vi "provePilot.vi"(8 "error in":errorcluster, 9 "Boiler Simulation Controls":refnum<vi>, 10 "Boiler Controls":refnum<vi>, 11 "Boiler Status Indicators":refnum<vi>) -> (0 "error out":errorcluster, 3 "sensor":dbl)   [LabVIEW 2024]
uses:
  Controls/Boiler Simulation Controls.ctl
  Controls/Boiler Status Indicators.ctl
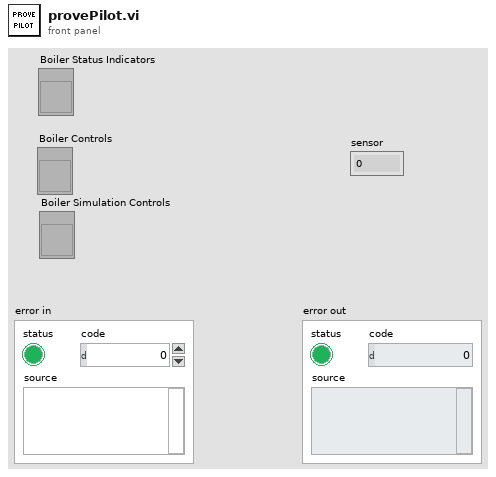
[diagram p1: front panel]
types:
  T1 = typedef "Boiler Simulation Controls.ctl" = cluster{"Flame Sensor Value (%)":dbl, "Run Interlock":bool, "Forced Draft Fan":bool}
  T2 = typedef "Boiler Status Indicators.ctl" = cluster{"Status":string, "Primary Fan":bool, "Natural Gas Valve":bool, "Pilot":bool, "Fuel Valve":bool, "Forced Draft Fan":bool, "Time Count":dbl}
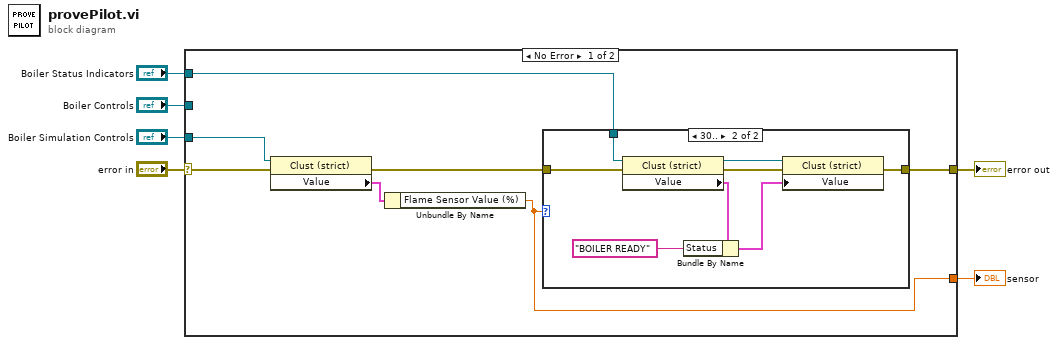
[diagram p0: block diagram]
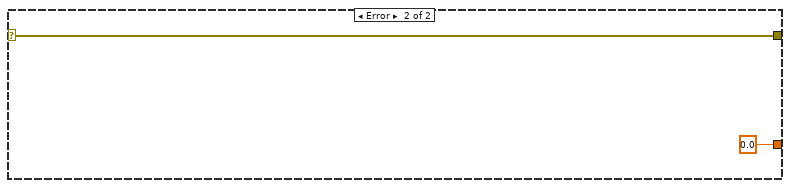
[diagram p3: hidden frame]
diagram:
  n1 = case shown="No Error" "error in" {
    selector: "error in" -> [w12 w24]
    tunnel: [w8 w24] -> w5
    tunnel: "Boiler Status Indicators" -> [w13 _]
    tunnel: [w7 0.0] -> w3
    tunnel: "Boiler Controls" -> [_ _]
    tunnel: "Boiler Simulation Controls" -> [w10 _]
    frame No Error {
      n2 = property class="Clust (strict)"(reference=w10, error in=w12) -> (error out=w11:errorcluster, "Value"=w9:T1)  [unwired: 1 out]
      n3 = Unbundle By Name(w9) -> ("Flame Sensor Value (%)"=w7:dbl)
      n4 = case shown="30.." w7 {
        tunnel: w13 -> [_ w22]
        tunnel: [w14 w16] -> w8
        tunnel: w11 -> [w14 w15]
        frame 0, Default {
        }
        frame 30.. {
          n5 = property class="Clust (strict)"(reference=w22, error in=w15) -> (reference out=w21:refnum<vi>, error out=w20:errorcluster, "Value"=w19:T2)
          n6 = Bundle By Name(cluster=w19, "Status"="BOILER READY") -> (w18:T2)
          n7 = property class="Clust (strict)"(reference=w21, error in=w20, "Value"=w18) -> (error out=w16:errorcluster)  [unwired: 1 out]
        }
      }
    }
    frame Error {
    }
  }
  "error out" <- w5
  "sensor" <- w3
